vi "Execute.vi"(8 "Error In":errorcluster, 11 "Draw Frame In":refnum<class "Draw Frame.lvclass">) -> (0 "Error Out":errorcluster, 3 "Draw Frame Out":refnum<class "Draw Frame.lvclass">)   [LabVIEW 2021, in "Draw Frame.lvclass"]
uses:
  Draw Frame.lvclass
  C:/Git/MEMOSFET/myDashBoard/Source/RT/Process/Process.lvclass
  Private/Controls/State.ctl
  Process/Process.lvclass
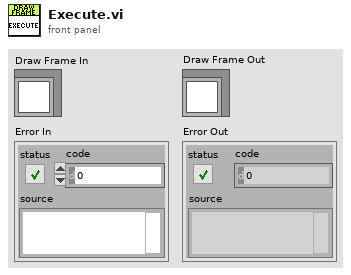
[diagram p1: front panel]
types:
  T1 = typedef "Draw Frame.lvclass/State.ctl" = enum16{"Initialize", "Wait for command", "Start Drawing", "Draw Frame", "Stop Drawing", "Shutdown"}
  T2 = typedef "Process.lvclass/Process Message.ctl" = cluster{"Command":string, "Data":variant}
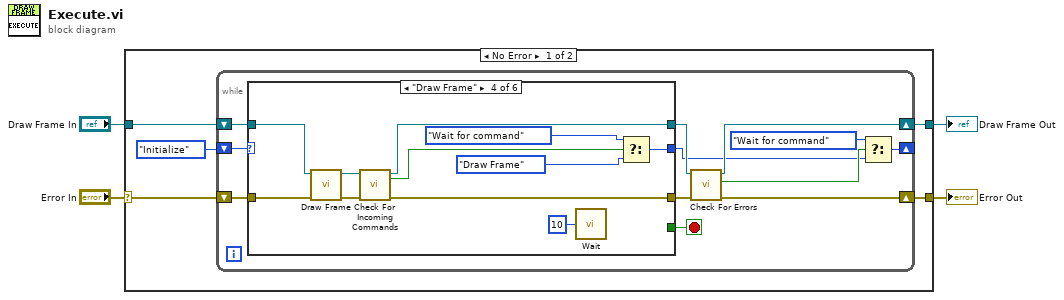
[diagram p0: block diagram]
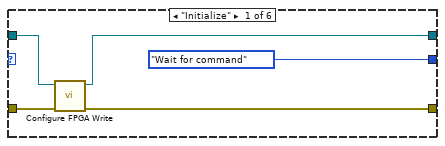
[diagram p2: hidden frame]
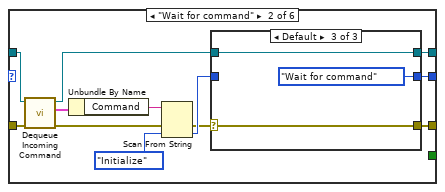
[diagram p3: hidden frame]
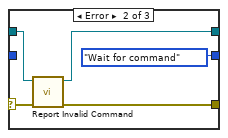
[diagram p5: hidden frame]
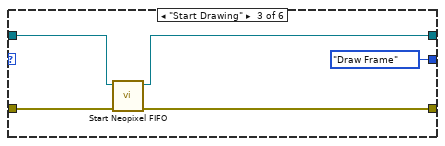
[diagram p6: hidden frame]
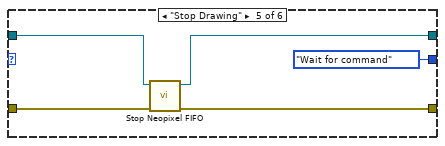
[diagram p7: hidden frame]
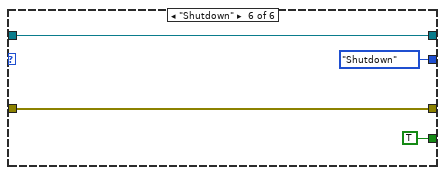
[diagram p8: hidden frame]
diagram:
  n1 = case shown="No Error" "Error In" {
    selector: "Error In" -> [w8 w76]
    tunnel: [w9 w76] -> w3
    tunnel: "Draw Frame In" -> [w6 w75]
    tunnel: [w5 w75] -> w1
    frame No Error {
      n2 = while {
        shift-right: [w17] -> w9
        shift-left: w8 -> [w21]
        shift-right: [w11] -> _
        shift-left: State."Initialize" ("State") -> [w20]
        shift-right: [w15] -> w5
        shift-left: w6 -> [w19]
        stop <- w14 stop-if-true
        n3 = case shown="\"Draw Frame\"" w20 {
          tunnel: w21 -> [w26 w37 w52 w65 w68 w72]
          tunnel: [w23 w27 w50 w60 w66 w72] -> w18
          tunnel: w19 -> [w25 w35 w53 w64 w69 w71]
          tunnel: [w24 w28 w51 w61 w67 w71] -> w16
          tunnel: [State."Wait for command" ("State") w29 State."Draw Frame" ("State") w56 State."Wait for command" ("State") State."Shutdown" ("State")] -> w12
          tunnel: [_ _ _ _ _ TRUE] -> w14
          frame "Initialize" {
            n4 = call "Configure FPGA Write.vi"("Error In"=w26, "Draw Frame In"=w25) -> ("Error Out"=w23:errorcluster, "Draw Frame Out"=w24:refnum<class "Draw Frame.lvclass">)  [unwired: 8 in]
          }
          frame "Wait for command" {
            n5 = call "Dequeue Incoming Command.vi"("Error In"=w37, "Process In"=w35) -> ("Error Out"=w31:errorcluster, "Process Message"=w36:T2, "Process Out"=w34:refnum<class "Draw Frame.lvclass">)  [unwired: 6 in, 1 out]
            n6 = Unbundle By Name(w36) -> ("Command"=w33:string)
            n7 = Scan From String(input string=w33, error in=w31, default 1=State."Initialize" ("State")) -> (error out=w30:errorcluster, output 1=w38:T1)  [unwired: 2 in, 2 out]
            n8 = case shown="Default" w30 {
              selector: w30 -> [w39 w44 w48]
              tunnel: w38 -> [w41 _ _]
              tunnel: [w41 State."Wait for command" ("State") State."Wait for command" ("State")] -> w29
              tunnel: w34 -> [w40 w46 w49]
              tunnel: [w40 w45 w49] -> w28
              tunnel: [w39 w43 w48] -> w27
              frame No Error {
              }
              frame Error {
                n9 = call "Report Invalid Command.vi"("Error In"=w44, "Process In"=w46) -> ("Error Out"=w43:errorcluster, "Process Out"=w45:refnum<class "Draw Frame.lvclass">)  [unwired: 8 in]
              }
              frame Default {
              }
            }
          }
          frame "Start Drawing" {
            n10 = call "Start Neopixel FIFO.vi"("Error In"=w52, "Draw Frame In"=w53) -> ("Error Out"=w50:errorcluster, "Draw Frame Out"=w51:refnum<class "Draw Frame.lvclass">)  [unwired: 8 in]
          }
          frame "Draw Frame" {
            n11 = call "Draw Frame.vi"("Error In"=w65, "Draw Frame In"=w64) -> ("Error Out"=w63:errorcluster, "Draw Frame Out"=w62:refnum<class "Draw Frame.lvclass">)  [unwired: 8 in]
            n12 = call "Check For Incoming Commands.vi"("Error In"=w63, "Process In"=w62) -> ("Error Out"=w60:errorcluster, "New Command(s)"=w59:bool, "Process Out"=w61:refnum<class "Draw Frame.lvclass">)  [unwired: 7 in]
            n13 = call "Wait"("Count(mSec)"=u32 10) -> ()  [unwired: 1 out]
            n14 = Select(t=State."Wait for command" ("State"), s=w59, f=State."Draw Frame" ("State")) -> (s? t:f=w56:T1)
          }
          frame "Stop Drawing" {
            n15 = call "Stop Neopixel FIFO.vi"("Error In"=w68, "Draw Frame In"=w69) -> ("Error Out"=w66:errorcluster, "Draw Frame Out"=w67:refnum<class "Draw Frame.lvclass">)  [unwired: 8 in]
          }
          frame "Shutdown" {
          }
        }
        n16 = call "Check For Errors.vi"("Error In"=w18, "Process In"=w16) -> ("Error Out"=w17:errorcluster, "Error Detected"=w13:bool, "Process Out"=w15:refnum<class "Draw Frame.lvclass">)  [unwired: 7 in]
        n17 = Select(t=State."Wait for command", s=w13, f=w12) -> (s? t:f=w11:T1)
      }
    }
    frame Error {
    }
  }
  "Error Out" <- w3
  "Draw Frame Out" <- w1
